vi "TCP Engine Close Active Engines.vi"(8 "error in":errorcluster, 11 "Engines Name":string[](array[string])) -> (0 "error out":errorcluster)   [LabVIEW 2024, in "TCP Engine.lvlib"]
doc: "All Rights Reserved © 2017 SyncSols"
uses:
  TCP Engine.lvlib
  Main Engine/Controls/Main Engine JSON Command State.ctl
  Analog Output/Controls/AIO Command Q Cluster.ctl
  Analog Output/Controls/AO Interface Data Cluster.ctl
  Analog Output/Controls/AO Channel Configuration Cluster.ctl
  Analog Output/Controls/AO Timing Cluster.ctl
  Digital Output/Controls/DIO Commad Q Cluster.ctl
  Digital Output/SubVIs/Digital Dynamic Cluster.ctl
  Async Serial/Controls/Async Serial Command Q Cluster.ctl
  Async Serial/Controls/Async Serial Configuration Cluster.ctl
  Async Serial/Controls/Async Frame Info Cluster.ctl
  Async Serial/Controls/Async Message Info Cluster.ctl
  Ethernet/Controls/Ethernet Command Q Cluster.ctl
  Ethernet/Controls/Ethernet Configuration Cluster.ctl
  Ethernet/Controls/Ethernet Frame Info Cluster.ctl
  Ethernet/Controls/Ethernet Message Info Cluster.ctl
  Ethernet/Controls/Ethernet Dynamic Data Cluster.ctl
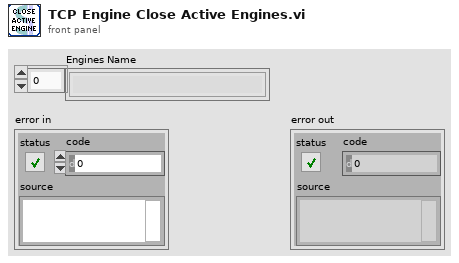
[diagram p1: front panel]
types:
  T1 = typedef "Main Engine JSON Command State.ctl" = enum16{"Configure", "Start", "Exit"}
  T2 = typedef "AIO Command Q Cluster.ctl" = cluster{"Interface":string, "Interface Data":T3, "Command State":T1}
  T3 = typedef "AO Interface Data Cluster.ctl" = cluster{"Command":string, "SubCmd":string, "Data":T4[], "Timing":T5}
  T4 = typedef "AO Channel Configuration Cluster.ctl" = cluster{"Channel":string, "Min Value":dbl, "Max Value":dbl, "Type":string, "Terminal Configure":u16, "Dynamic":u8, "Dyn Type":string, "Data":dbl[], "File Name":string, "Column":i32, "Frequency":dbl}
  T5 = typedef "AO Timing Cluster.ctl" = cluster{"samples per channel":i32, "sample mode":i32, "Sampling Rate":dbl}
  T6 = typedef "DIO Commad Q Cluster.ctl" = cluster{"Interface":string, "Interface Data":cluster{"Command":string, "SubCmd":string, "Frequency":u16, "Data":T7[]}, "Command State":T1}
  T7 = typedef "Digital Dynamic Cluster.ctl" = cluster{"Channel":string, "Data":u8[], "Identification Name":string}
  T8 = typedef "Async Serial Command Q Cluster.ctl" = cluster{"Async serial Configuration Cluster":T9, "Command State":T1}
  T9 = typedef "Async Serial Configuration Cluster.ctl" = cluster{"Port":string, "Minor Frame Freq":u16, "Minor Frame Count":u16, "Frame Info":T10[], "Sensor Type":u16, "OIM Address":u16}
  T10 = typedef "Async Frame Info Cluster.ctl" = cluster{"Frame ID":u16, "Message Info":T11[]}
  T11 = typedef "Async Message Info Cluster.ctl" = cluster{"Message":u8[], "Message Name":string}
  T12 = typedef "Ethernet Command Q Cluster.ctl" = cluster{"Ethernet Configuration":T13, "Command State":T1}
  T13 = typedef "Ethernet Configuration Cluster.ctl" = cluster{"Mode":u8, "Local IP":string, "Local Port":u16, "Frame Info":T14[], "Minor Frame Freq":u8}
  T14 = typedef "Ethernet Frame Info Cluster.ctl" = cluster{"Frame ID":u16, "Message Info":T15[]}
  T15 = typedef "Ethernet Message Info Cluster.ctl" = cluster{"Message":u8[], "Message Name":string, "Dynamic":u8, "DynData":T16[], "Client IP":string, "Client Port":u16}
  T16 = typedef "Ethernet Dynamic Data Cluster.ctl" = cluster{"Type":string, "Start Byte":u8, "End Byte":u8, "Data":u32[][], "File Name":string, "Column":i32}
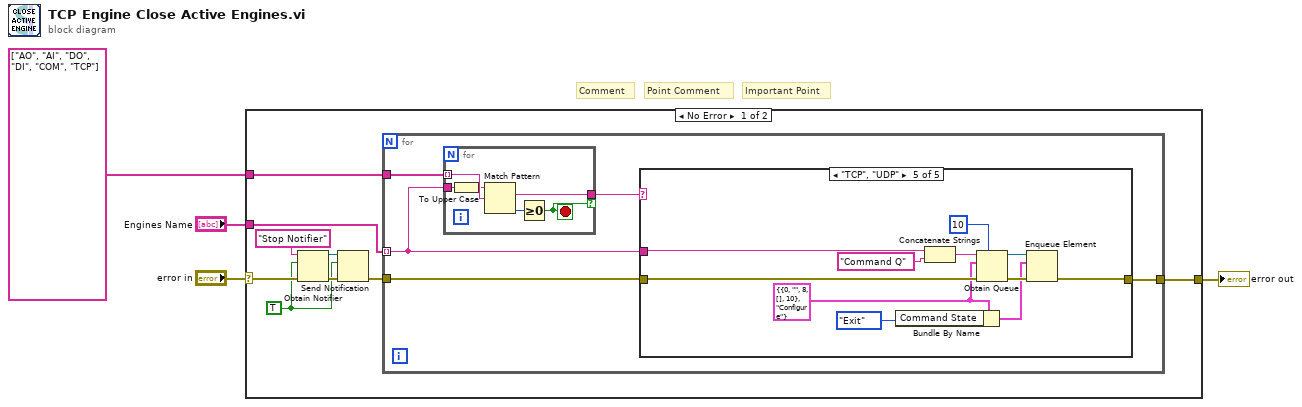
[diagram p0: block diagram]
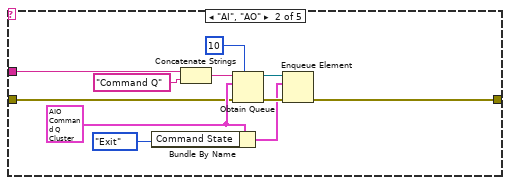
[diagram p3: hidden frame]
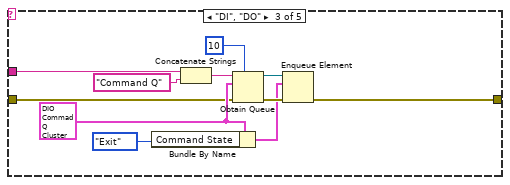
[diagram p4: hidden frame]
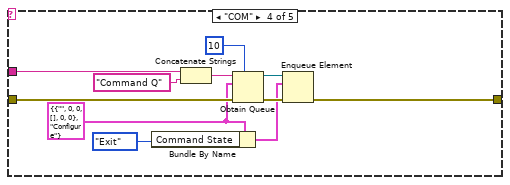
[diagram p5: hidden frame]
diagram:
  # "Important Point"
  # "Point Comment"
  # "Comment"
  n1 = case shown="No Error" "error in" {
    selector: "error in" -> [w10 w70]
    tunnel: [w12 w70] -> w4
    tunnel: "Engines Name" -> [w13 _]
    tunnel: string[] ["AO", "AI", "DO", "DI", "COM", "TCP"] -> [w11 _]
    frame No Error {
      w5 = TRUE
      n2 = Obtain Notifier(name (unnamed)="Stop Notifier", notification data type=w5, error in (no error)=w10) -> (notifier out=w6:refnum<notifier>, error out=w9:errorcluster)  [unwired: 1 in, 1 out]
      n3 = Send Notification(notification=w5, notifier=w6, error in (no error)=w9) -> (error out=w8:errorcluster)  [unwired: 1 out]
      n4 = for {
        tunnel: w13 -> [w15] mode=indexing
        tunnel: w8 -> [w18]
        tunnel: [w17] -> w12
        tunnel: w11 -> [w16]
        n5 = for {
          tunnel: w16 -> [w23] mode=indexing
          tunnel: w15 -> [w24]
          tunnel: [w21] -> w14 if=w20
          stop <- w20 stop-if-true
          n6 = To Upper Case(1:w24) -> (0:w19:string)
          n7 = Match Pattern(string=w19, regular expression=w23) -> (match substring=w21:string, offset past match=w22:i32)  [unwired: 1 in, 2 out]
          n8 = Greater Or Equal To 0?(x=w22) -> (x >= 0?=w20:bool)
        }
        n9 = case shown="\"TCP\", \"UDP\"" w14 {
          tunnel: w15 -> [_ w30 w41 w52 w60]
          tunnel: w18 -> [w25 w28 w39 w51 w62]
          tunnel: [w25 w27 w38 w50 w61] -> w17
          frame "False", Default {
          }
          frame "AI", "AO" {
            w29 = T2 {"Interface"="AIO", "Interface Data"={"Command"="Configure", "SubCmd"="AO", "Data"=[], "Timing"={"samples per channel"=1000, "sample mode"=10178, "Sampling Rate"=1000.0}}, "Command State"=enum."Configure"}
            n10 = Bundle By Name(cluster=w29, "Command State"=Main_Engine_JSON_Command_State."Exit") -> (w31:T2)
            n11 = Concatenate Strings(w30, "Command Q" ("string")) -> (w34:string)
            n12 = Obtain Queue(max queue size (-1, unlimited)=10, name (unnamed)=w34, element data type=w29, error in (no error)=w28) -> (queue out=w33:refnum<queue>, error out=w36:errorcluster)  [unwired: 1 in, 1 out]
            n13 = Enqueue Element(queue=w33, element=w31, error in (no error)=w36) -> (error out=w27:errorcluster)  [unwired: 1 in, 2 out]
          }
          frame "DI", "DO" {
            w40 = T6 {"Interface"="AIO", "Interface Data"={"Command"="Configure", "SubCmd"="AO", "Frequency"=0, "Data"=[]}, "Command State"=enum."Configure"}
            n14 = Bundle By Name(cluster=w40, "Command State"=Main_Engine_JSON_Command_State."Exit") -> (w42:T6)
            n15 = Concatenate Strings(w41, "Command Q" ("string")) -> (w45:string)
            n16 = Obtain Queue(max queue size (-1, unlimited)=10, name (unnamed)=w45, element data type=w40, error in (no error)=w39) -> (queue out=w44:refnum<queue>, error out=w47:errorcluster)  [unwired: 1 in, 1 out]
            n17 = Enqueue Element(queue=w44, element=w42, error in (no error)=w47) -> (error out=w38:errorcluster)  [unwired: 1 in, 2 out]
          }
          frame "COM" {
            w48 = T8 {"Async serial Configuration Cluster"={"Port"="", "Minor Frame Freq"=0, "Minor Frame Count"=0, "Frame Info"=[], "Sensor Type"=0, "OIM Address"=0}, "Command State"=enum."Configure"} ("Async Serial Command Q Cluster")
            n18 = Bundle By Name(cluster=w48, "Command State"=Main_Engine_JSON_Command_State."Exit") -> (w53:T8)
            n19 = Concatenate Strings(w52, "Command Q" ("string")) -> (w56:string)
            n20 = Obtain Queue(max queue size (-1, unlimited)=10, name (unnamed)=w56, element data type=w48, error in (no error)=w51) -> (queue out=w55:refnum<queue>, error out=w58:errorcluster)  [unwired: 1 in, 1 out]
            n21 = Enqueue Element(queue=w55, element=w53, error in (no error)=w58) -> (error out=w50:errorcluster)  [unwired: 1 in, 2 out]
          }
          frame "TCP", "UDP" {
            w59 = T12 {"Ethernet Configuration"={"Mode"=0, "Local IP"="", "Local Port"=8, "Frame Info"=[], "Minor Frame Freq"=10}, "Command State"=enum."Configure"} ("Async Serial Command Q Cluster")
            n22 = Bundle By Name(cluster=w59, "Command State"=Main_Engine_JSON_Command_State."Exit") -> (w64:T12)
            n23 = Concatenate Strings(w60, "Command Q" ("string")) -> (w67:string)
            n24 = Obtain Queue(max queue size (-1, unlimited)=10, name (unnamed)=w67, element data type=w59, error in (no error)=w62) -> (queue out=w66:refnum<queue>, error out=w69:errorcluster)  [unwired: 1 in, 1 out]
            n25 = Enqueue Element(queue=w66, element=w64, error in (no error)=w69) -> (error out=w61:errorcluster)  [unwired: 1 in, 2 out]
          }
        }
      }
    }
    frame Error {
    }
  }
  "error out" <- w4
